vi "版本号读取.vi"(7 "是否启用通讯通知":bool, 8 "error in (no error)":errorcluster, 11 "Slave ID":T1) -> (0 "error out":errorcluster, 3 "固件信息":string)   [LabVIEW 2016, in "质控单元V1.lvlib"]
uses:
  <vilib>/Plasmionique/MB Master/MB_Master/MB_Master.lvclass
  <vilib>/Plasmionique/MB Master/MB Master.lvlib
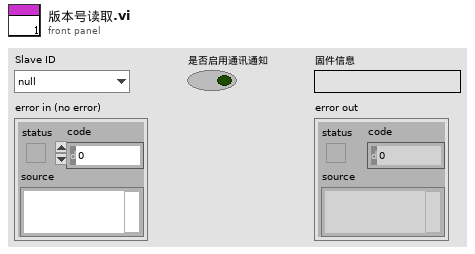
[diagram p1: front panel]
types:
  T1 = typedef "质控单元V1.lvlib/质控slave id.ctl" = enum16{"null", "氨氮", "总磷", "CODMn", "CODCr", "总氮"}
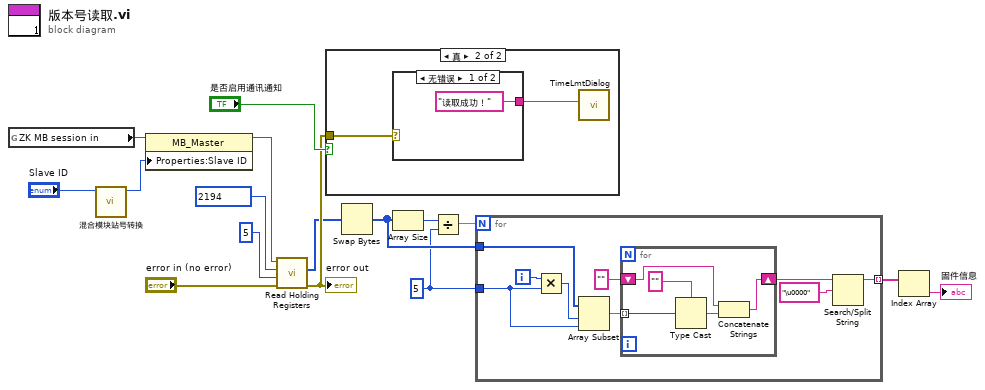
[diagram p0: block diagram]
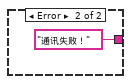
[diagram p3: hidden frame]
diagram:
  w5 = 5 ("字符个数")
  n1 = global read "ZK非断电保存全局变量.vi" "ZK MB session in"() -> (w15:refnum<class "MB_Master.lvclass">)
  n2 = call "混合模块站号转换.vi"("Slave ID输入"="Slave ID") -> ("Slave ID输出"=w1:T1)  [unwired: 10 in]
  n3 = property class="MB_Master"(reference=w15, "Properties:Slave ID"=w1) -> (reference out=w13:refnum<class "MB_Master.lvclass">)  [unwired: 1 in, 1 out]
  n4 = call <vilib>:"Read Holding Registers.vi"("error in (no error)"="error in (no error)", "quantity"=u16 5, "starting address"=u16 2194, "MB session in"=w13) -> ("error out"=w10:errorcluster, "Registers"=w6:u16[])  [unwired: 5 in, 1 out]
  "error out" <- w10
  n5 = case shown="真" "是否启用通讯通知" {
    tunnel: w10 -> [_ w18]
    frame False {
    }
    frame True {
      n6 = case shown="无错误" w18 {
        tunnel: ["读取成功！" "通讯失败！"] -> w17
        frame No Error {
        }
        frame Error {
        }
      }
      n7 = call "TimeLmtDialog.vi"("Infoin"=w17) -> ()  [unwired: 11 in]
    }
  }
  n8 = Swap Bytes(anything=w6) -> (byte swapped=w7:u16[])
  n9 = Array Size(array=w7) -> (size(s)=w9:i32)
  n10 = Divide(x=w9, y=w5) -> (x/y=w8:dbl)
  n11 = for {
    N: w8 -> [_]
    tunnel: w7 -> [w29]
    tunnel: [w23] -> w4 mode=indexing
    tunnel: w5 -> [w22]
    i -> [w28]
    n12 = Multiply(x=w28, y=w22) -> (x*y=w27:i32)
    n13 = Array Subset(array=w29, index=w27, length=w22) -> (w25:u16[])
    n14 = for {
      shift-right: [w34] -> w24
      shift-left: "" -> [w31]
      tunnel: w25 -> [w33] mode=indexing
      n15 = Type Cast(type="", x=w33) -> (*(type *) &x=w30:string)
      n16 = Concatenate Strings(w31, w30) -> (w34:string)
    }
    n17 = Search/Split String(string=w24, search string/char (-)="\u0000" ("搜索字符串")) -> (substring before match=w23:string)  [unwired: 1 in, 2 out]
  }
  n18 = Index Array(array=w4) -> (element=→"固件信息":string)  [unwired: 1 in]
